vi "refNewton Raphson Inner Part user defined derivative.vi"(4 "accuracy":dbl format="%.2f", 5 "end/start":dbl format="%.2f", 6 "case":bool, 7 "start/end":dbl format="%.2f", 9 "Variant":variant, 10 "function refnum":T1) -> (0 "error":i32, 1 "f'(zero)":dbl, 2 "zero":dbl format="%.2f", 3 "f(zero)":dbl format="%.2f")   [LabVIEW 2017, in "NI_Gmath.lvlib"]
uses:
  <vilib>/gmath/NI_Gmath.lvlib
  <vilib>/gmath/_ref_NR.llb/functionAndDerivativeRefnum.ctl
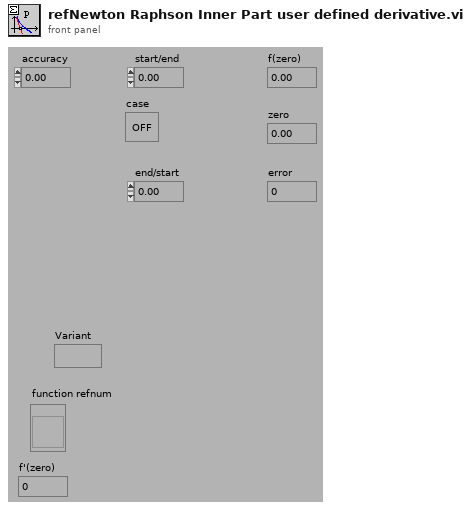
[diagram p1: front panel]
types:
  T1 = typedef "NI_Gmath.lvlib/functionAndDerivativeRefnum.ctl" = refnum<vi>
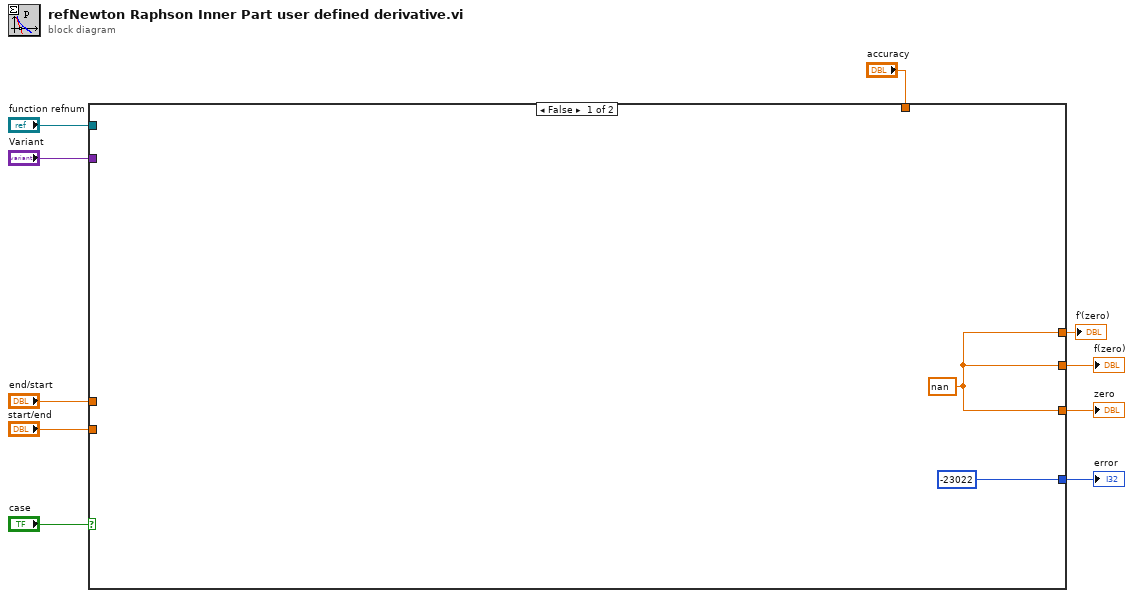
[diagram p0: block diagram]
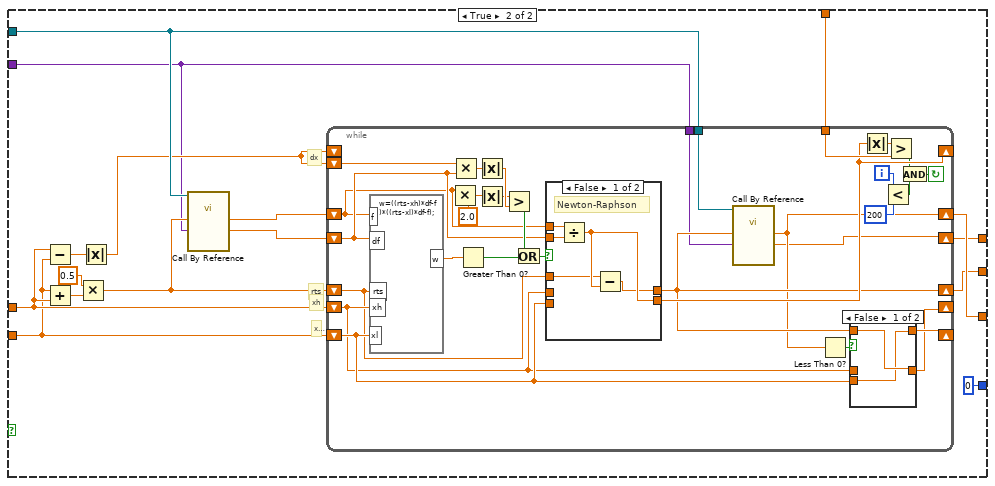
[diagram p2: hidden frame]
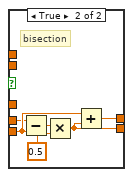
[diagram p4: hidden frame]
diagram:
  n1 = case shown="False" "case" {
    tunnel: [w11 w27] -> w5
    tunnel: [w11 w26] -> w4
    tunnel: "end/start" -> [_ w25]
    tunnel: "start/end" -> [_ w24]
    tunnel: "accuracy" -> [_ w21]
    tunnel: [-23022 0] -> w8
    tunnel: "function refnum" -> [_ w28]
    tunnel: "Variant" -> [_ w13]
    tunnel: [w11 w17] -> w1
    frame False {
      w11 = nan
    }
    frame True {
      # "rts"
      # "dx"
      # "xh"
      # "xl"
      n2 = Subtract(x=w25, y=w24) -> (x-y=w23:dbl)
      n3 = Add(x=w24, y=w25) -> (x+y=w19:dbl)
      n4 = Multiply(x=0.5, y=w19) -> (x*y=w14:dbl)
      n5 = Absolute Value(x=w23) -> (abs(x)=w22:dbl)
      n6 = call-by-ref "?"(reference=w28, "Variant"=w13, "x"=w14) -> ("f'(x)"=w15:dbl, "f(x)"=w16:dbl)  [unwired: 3 in, 2 out]
      n7 = while {
        tunnel: w21 -> [w43]
        shift-left: w22 -> [w42]
        shift-left: w24 -> [w49]
        shift-right: [w47] -> _
        shift-left: w25 -> [w48]
        shift-right: [w46] -> _
        shift-left: w15 -> [w51]
        shift-right: [w29] -> w17
        shift-left: w16 -> [w45]
        shift-right: [w30] -> w27
        shift-left: w22 -> [_]
        shift-right: [w39] -> _
        shift-left: w14 -> [w44]
        shift-right: [w32] -> w26
        tunnel: w28 -> [w58]
        tunnel: w13 -> [w31]
        i -> [w37]
        stop <- w33 continue-if-true
        n8 = formula code="w=((rts-xh)*df-f)*((rts-xl)*df-f);"("f"=w45, "df"=w51, "rts"=w44, "xh"=w48, "xl"=w49) -> ("w"=w38:dbl)
        n9 = Multiply(x=w45, y=2.0) -> (x*y=w55:dbl)
        n10 = Multiply(x=w42, y=w51) -> (x*y=w56:dbl)
        n11 = Greater Than 0?(x=w38) -> (x > 0?=w40:bool)
        n12 = Absolute Value(x=w56) -> (abs(x)=w59:dbl)
        n13 = Absolute Value(x=w55) -> (abs(x)=w54:dbl)
        n14 = Greater?(x=w54, y=w59) -> (0:w53:bool)
        n15 = Or(x=w53, y=w40) -> (x .or. y?=w52:bool)
        n16 = case shown="False" w52 {
          tunnel: w48 -> [_ w73]
          tunnel: w49 -> [_ w74]
          tunnel: [w68 w70] -> w39
          tunnel: [w64 w69] -> w32
          tunnel: w45 -> [w67 _]
          tunnel: w51 -> [w66 _]
          tunnel: w44 -> [w65 _]
          frame False {
            # "Newton-Raphson"
            n17 = Divide(x=w67, y=w66) -> (x/y=w68:dbl)
            n18 = Subtract(x=w65, y=w68) -> (x-y=w64:dbl)
          }
          frame True {
            # "bisection"
            n19 = Subtract(x=w73, y=w74) -> (x-y=w72:dbl)
            n20 = Multiply(x=w72, y=0.5) -> (x*y=w70:dbl)
            n21 = Add(x=w74, y=w70) -> (x+y=w69:dbl)
          }
        }
        n22 = call-by-ref "?"(reference=w58, "Variant"=w31, "x"=w32) -> ("f'(x)"=w29:dbl, "f(x)"=w30:dbl)  [unwired: 3 in, 2 out]
        n23 = Less Than 0?(x=w30) -> (x < 0?=w50:bool)
        n24 = case shown="False" w50 {
          tunnel: w49 -> [w60 _]
          tunnel: w48 -> [_ w62]
          tunnel: w32 -> [w61 w63]
          tunnel: [w60 w63] -> w47
          tunnel: [w61 w62] -> w46
          frame False {
          }
          frame True {
          }
        }
        n25 = Absolute Value(x=w39) -> (abs(x)=w41:dbl)
        n26 = Less?(x=w37, y=200) -> (x < y?=w35:bool)
        n27 = Greater?(x=w41, y=w43) -> (0:w34:bool)
        n28 = And(x=w34, y=w35) -> (x .and. y?=w33:bool)
      }
    }
  }
  "error" <- w8
  "zero" <- w5
  "f(zero)" <- w4
  "f'(zero)" <- w1
